vi "getFile TestID.vi"(8 "error in (no error)":errorcluster, 11 "Path":path=path "C:/Users/Flash/Documents/GitHub/labview/Detector IV/rawtest_log.csv") -> (0 "error out":errorcluster, 3 "TestID":u32=1995)   [LabVIEW 2012]
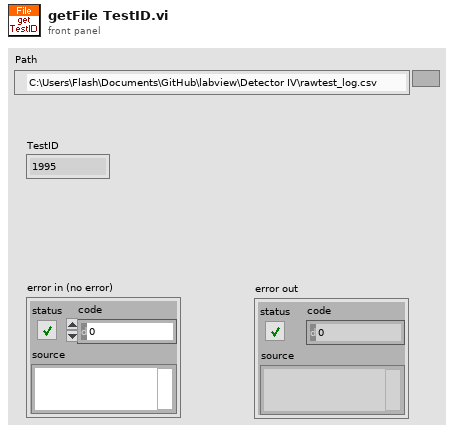
[diagram p1: front panel]
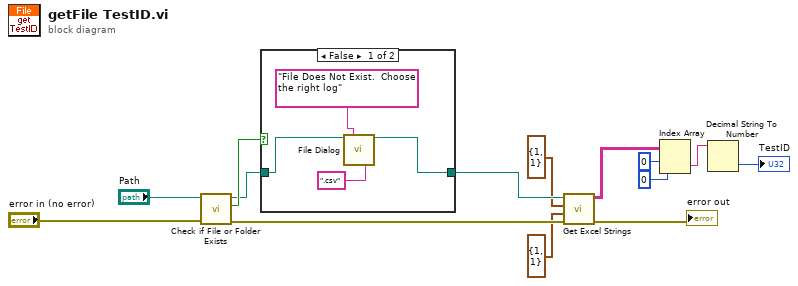
[diagram p0: block diagram]
diagram:
  n1 = call <vilib>:"Check if File or Folder Exists.vi"("error in (no error)"="error in (no error)", "path"="Path") -> ("error out"=w9:errorcluster, "file or folder exists?"=w12:bool, "dup path"=w11:path)  [unwired: 7 in]
  n2 = case shown="False" w12 {
    tunnel: w11 -> [w18 w19]
    tunnel: [w17 w19] -> w10
    frame False {
      n3 = call "File Dialog"("start path"=w18, "prompt"="File Does Not Exist.  Choose the right log", "pattern label"=".csv") -> ("selected path"=w17:path)  [unwired: 9 in, 3 out]
    }
    frame True {
    }
  }
  n4 = call "Get Excel Strings.vi"("error in (no error)"=w9, "End"=cluster{"Column":i32, "Row":i32} {"Column"=1, "Row"=1}, "Start"=cluster{"Column":i32, "Row":i32} {"Column"=1, "Row"=1}, "path"=w10) -> ("error out"=→"error out":errorcluster, "data"=w5:string[][])  [unwired: 1 in, 5 out]
  n5 = Index Array(array=w5, index (row)=0, index (col)=0 ("disabled index (col)")) -> (element=w2:string)
  n6 = Decimal String To Number(string=w2) -> (number=→"TestID":i32)  [unwired: 2 in, 1 out]
